vi "testLedBlink.vi"() -> ()   [LabVIEW 2019]
doc: "Tests the method blinkLED"
uses:
  3bc6ffe6-1ab6-43e8-9219-b4bcd59879eb.vi
  LED Class/LED.lvclass
panel:
  out "Yellow":bool
  out "Green":bool
  out "Red":bool
  out "Blue":bool
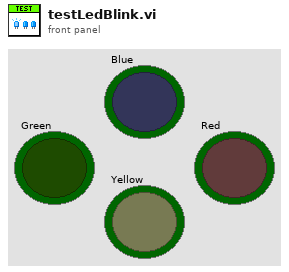
[diagram p1: front panel]
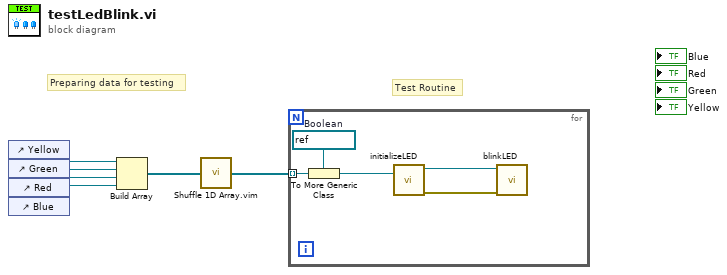
[diagram p0: block diagram]
diagram:
  # "Test Routine"
  # "Preparing data for testing"
  n1 = control-ref of="Yellow"() -> (w6:refnum<vi>)
  n2 = control-ref of="Green"() -> (w5:refnum<vi>)
  n3 = control-ref of="Red"() -> (w4:refnum<vi>)
  n4 = control-ref of="Blue"() -> (w3:refnum<vi>)
  n5 = Build Array(w6, w5, w4, w3) -> (w2:refnum<vi>[])
  n6 = call "Shuffle 1D Array.vim"("array"=w2) -> ("shuffled array"=w1:refnum<vi>[])  [unwired: 4 in]
  n7 = for {
    tunnel: w1 -> [w9] mode=indexing
    w7 = refnum<vi> refnum  # Boolean
    n8 = To More Generic Class(target class=w7, reference=w9) -> (generic class reference=w8:refnum<vi>)
    n9 = call "initializeLED.vi"("LED Refnum"=w8) -> ("error out"=w10:errorcluster, "LED out"=w11:refnum<class "LED.lvclass">)  [unwired: 9 in]
    n10 = call "blinkLED.vi"("error in (no error)"=w10, "LED in"=w11) -> ()  [unwired: 8 in, 2 out]
  }
